vi "get pid array.vi"(8 "error in (no error)":errorcluster, 11 "Array in":T2) -> (0 "error out":errorcluster, 2 "Value":T1[](array[typedef]), 3 "Array out":T2)   [LabVIEW 2013, in "PID Module editor node.lvclass"]
uses:
  PID Module editor node.lvclass
  PID array reference.ctl
  PID array element.ctl
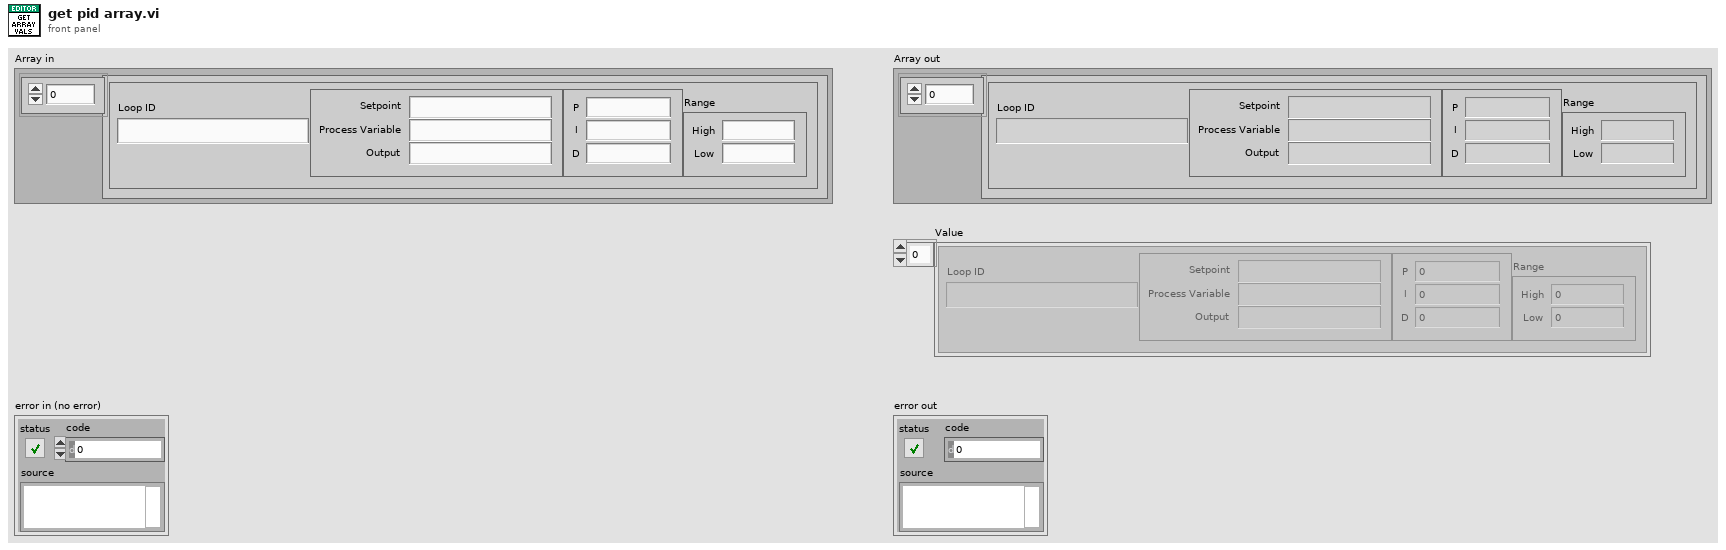
[diagram p1: front panel]
types:
  T1 = typedef "PID Module editor node.lvclass/PID array element.ctl" = cluster{"Loop ID":string, "Tags":cluster{"Setpoint":string, "Process Variable":string, "Output":string}, "Gains":cluster{"P":dbl, "I":dbl, "D":dbl}, "Range":cluster{"High":dbl, "Low":dbl}}
  T2 = typedef "PID Module editor node.lvclass/PID array reference.ctl" = refnum<vi>
  T3 = typedef "Tagbus PID Module editor node.lvclass/PID array element.ctl" = cluster{"Loop ID":string, "Tags":cluster{"Setpoint":string, "Process Variable":string, "Output":string}, "Gains":cluster{"P":dbl, "I":dbl, "D":dbl}, "Range":cluster{"High":dbl, "Low":dbl}}
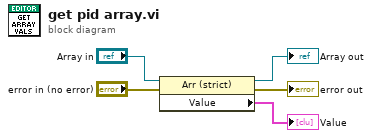
[diagram p0: block diagram]
diagram:
  n1 = property class="Arr (strict)"(reference="Array in", error in="error in (no error)") -> (reference out=→"Array out":T2, error out=→"error out":errorcluster, "Value"=→"Value":T3[])
